vi "BGA244_set_gas_type.vi"(8 "error in":errorcluster, 9 "gas 2":string, 10 "gas 1":string, 11 "VISA in":refnum<visa-resource-name>) -> (0 "error out":errorcluster, 3 "VISA out":refnum<visa-resource-name>, 4 "status":bool)   [LabVIEW 2019]
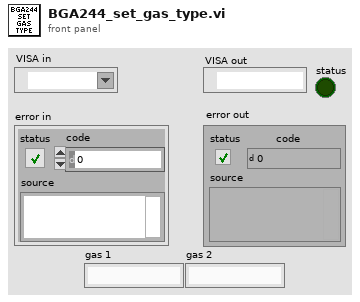
[diagram p1: front panel]
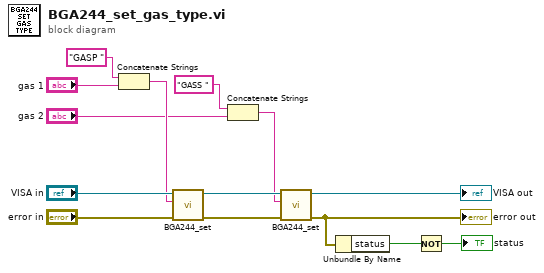
[diagram p0: block diagram]
diagram:
  n1 = Concatenate Strings("GASP " ("string"), "gas 1") -> (w4:string)
  n2 = call "BGA244_set.vi"("error in"="error in", "string in"=w4, "VISA in"="VISA in") -> ("error out"=w10:errorcluster, "VISA out"=w12:refnum<visa-resource-name>)  [unwired: 7 in]
  n3 = Concatenate Strings("GASS " ("string"), "gas 2") -> (w1:string)
  n4 = call "BGA244_set.vi"("error in"=w10, "string in"=w1, "VISA in"=w12) -> ("error out"=w9:errorcluster, "VISA out"=→"VISA out":refnum<visa-resource-name>)  [unwired: 7 in]
  "error out" <- w9
  n5 = Unbundle By Name(w9) -> ("status"=w8:bool)
  n6 = Not(x=w8) -> (.not. x?=→"status":bool)
